vi "Open.vi"(8 "error in (no error)":errorcluster, 9 "Worksheet Name (Sheet1)":string="Sheet1", 10 "File Path":path, 11 "Excel in":refnum<class "Excel.lvclass">) -> (0 "error out":errorcluster, 3 "Excel out":refnum<class "Excel.lvclass">)   [LabVIEW 2016, in "Excel.lvclass"]
doc: "Opens Excel, a workbook, and a sheet within that workbook.\n\nIf an Excel application is already running the existing instance is used. If it is not running a new instance is started.\n\nIf a file path is provided the workbook at that path will be opened. If a file path is not provided but this Excel object has previously opened a workbook that workbook will be opened. If a file path is not provided and no workbook has been previously been opened the user will be prompted to either make a new workbook, open an existing workbook, or use the currently active workbook.\n\nIf a worksheet name is provided that sheet will be activated and shown within the workbook. If the worksheet does not exist within the workbook it will be created. If no sheet name is specified a default \"Sheet1\" is used and will also be created if not found in the workbook."
uses:
  Excel.lvclass
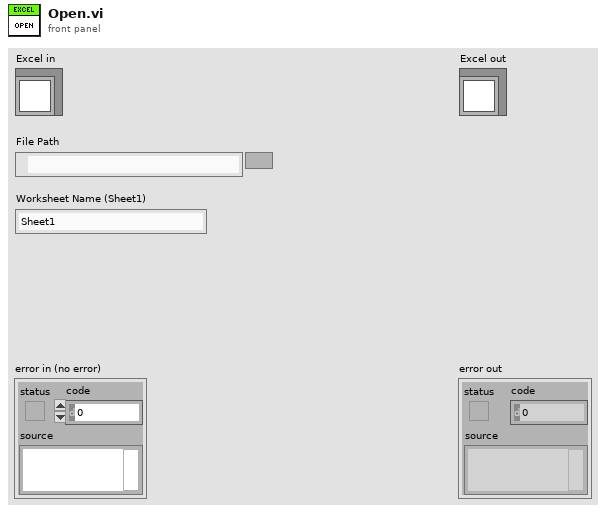
[diagram p1: front panel]
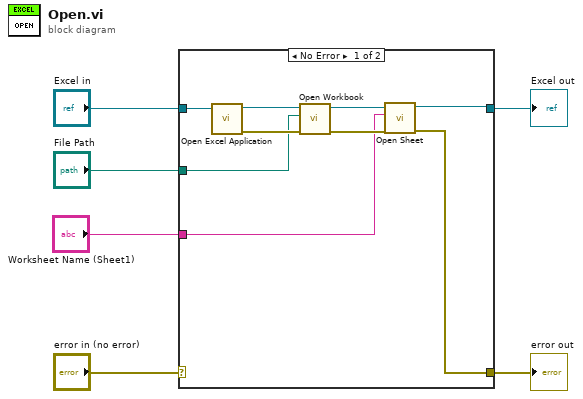
[diagram p0: block diagram]
diagram:
  n1 = case shown="No Error" "error in (no error)" {
    selector: "error in (no error)" -> [_ w17]
    tunnel: [w7 w17] -> w5
    tunnel: [w8 w16] -> w3
    tunnel: "Excel in" -> [w15 w16]
    tunnel: "File Path" -> [w12 _]
    tunnel: "Worksheet Name (Sheet1)" -> [w9 _]
    frame No Error {
      n2 = call "Open Excel Application.vi"("Excel in"=w15) -> ("Excel out"=w14:refnum<class "Excel.lvclass">, "error out"=w13:errorcluster)  [unwired: 8 in]
      n3 = call "Open Workbook.vi"("error in (no error)"=w13, "File Path (last path)"=w12, "Excel in"=w14) -> ("error out"=w10:errorcluster, "Excel out"=w11:refnum<class "Excel.lvclass">)  [unwired: 7 in]
      n4 = call "Open Sheet.vi"("error in (no error)"=w10, "Name (Sheet1)"=w9, "Excel in"=w11) -> ("error out"=w7:errorcluster, "Excel out"=w8:refnum<class "Excel.lvclass">)  [unwired: 7 in]
    }
    frame Error {
    }
  }
  "error out" <- w5
  "Excel out" <- w3
